vi "ToolBarButtonDraw.vi"(8 "error in (no error)":errorcluster, 9 "Coords":T1, 11 "Gviewer in":refnum<class "Gviewer.lvclass">) -> (0 "error out":errorcluster, 3 "Gviewer out":refnum<class "Gviewer.lvclass">)   [LabVIEW 2020, in "Sgraph_lib_V1.lvlib" / "Gviewer.lvclass"]
doc: "Draw toolbar buttons and objects on mouse move"
uses:
  Gviewer.lvclass
  <vilib>/Utility/miscctls.llb/LVPoint32TypeDef.ctl
  Gviewer.lvclass/Gviewer.ctl
  controls/AutoScale.ctl
  Common/controls/ToolTypeEnum.ctl
  Builds/Sgraph_lib_V1.lvlib
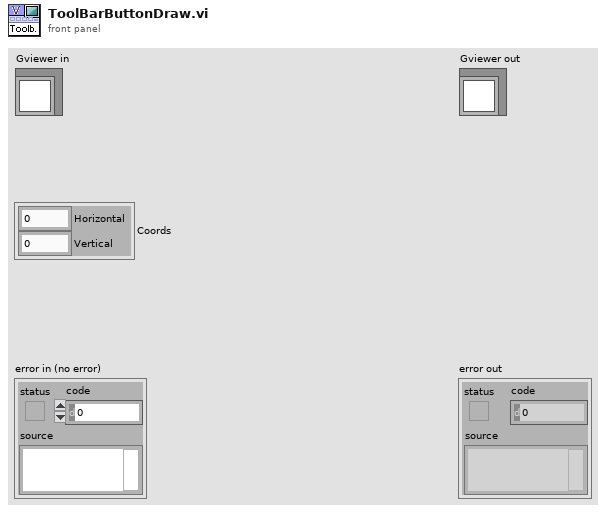
[diagram p1: front panel]
types:
  T1 = typedef "LVPoint32TypeDef.ctl" = cluster{"Horizontal":i32, "Vertical":i32}
  T2 = cluster{"left":i16, "top":i16, "right":i16, "bottom":i16}
  T3 = cluster{"horizontal":enum16{"left", "center", "right"}, "vertical":enum16{"top", "center", "bottom"}}
  T4 = typedef "Sgraph_lib_V1.lvlib/Gviewer.lvclass/AutoScale.ctl" = enum16{"FitEqual", "FitMax", "StackEqual", "StackMax", "StackPerType"}
  T5 = typedef "Sgraph_lib_V1.lvlib/Gviewer.lvclass/Typedef_ZoomEvent.ctl" = cluster{"Time-Start":timestamp, "Time-End":timestamp, "TimeSpan(sec)":dbl, "Live":T6, "SelProperties":T7[], "Time Stamp":timestamp}
  T6 = typedef "Sgraph_lib_V1.lvlib/Gviewer.lvclass/Typedef_Live.ctl" = enum16{"Live View", "Freeze"}
  T7 = typedef "Sgraph_lib_V1.lvlib/Gviewer.lvclass/Typedef_SelProperties.ctl" = cluster{"Color":u32, "LineType":T8, "max":dbl, "min":dbl}
  T8 = typedef "Sgraph_lib_V1.lvlib/Gviewer.lvclass/Typedef_LineType.ctl" = enum16{"num_bare", "num_MinMax_Area", "num_MinMax_Lines", "num_MinMax_Forfor", "num_Max_Area", "num_Max_Line", "num_Max_Forfor", "num_Min_Area", "num_Min_Line", "num_Min_Fosfor", "Boolean_Line_01", "Boolean_Area_01", "Boolean_Fosfor_01", "Boolean_Line_TF", "Boolean_Area_TF", "Boolean_Fosfor_TF", "Boolean_OnOff_Line", "Boolean_OnOff_Area", "Boolean_OnOff_Fosfor", "Boolean_spare", "StringEvent_Line", "StringEvent_TimeLine"}
  T9 = typedef "Sgraph_lib_V1.lvlib/ToolTypeEnum.ctl" = enum16{"00_Esc button", "01_Undo", "02_HelpButton", "03_CursorViewButton", "04_AutoScale_Fit", "05_AutoScale_Stacked", "06_ZoomWindowStart", "07_ZoomTimeStart", "08_ZoomAmplitudeStart", "09", "10", "11", "12", "13", "14", "15", "16", "17", "18", "19", "20_VerticalScroll", "21_VerticalMove", "22_TimeScroll", "23_TimeMove", "24", "25", "26_ZoomWindowSize", "27_ZoomTimeWindowSize", "28_ZoomAmplitudeWindowSize", "29", "30_LegendMovePoint", "31_LegendMoveDrag", "32", "33", "34", "35", "36", "37", "38", "39", "40_AddYscalePoint", "41_AddYscalePlace", "42_AddYscaleMovePoint", "43_AddYscaleMoveDrag", "44_AddYscaleDeletePoint"}
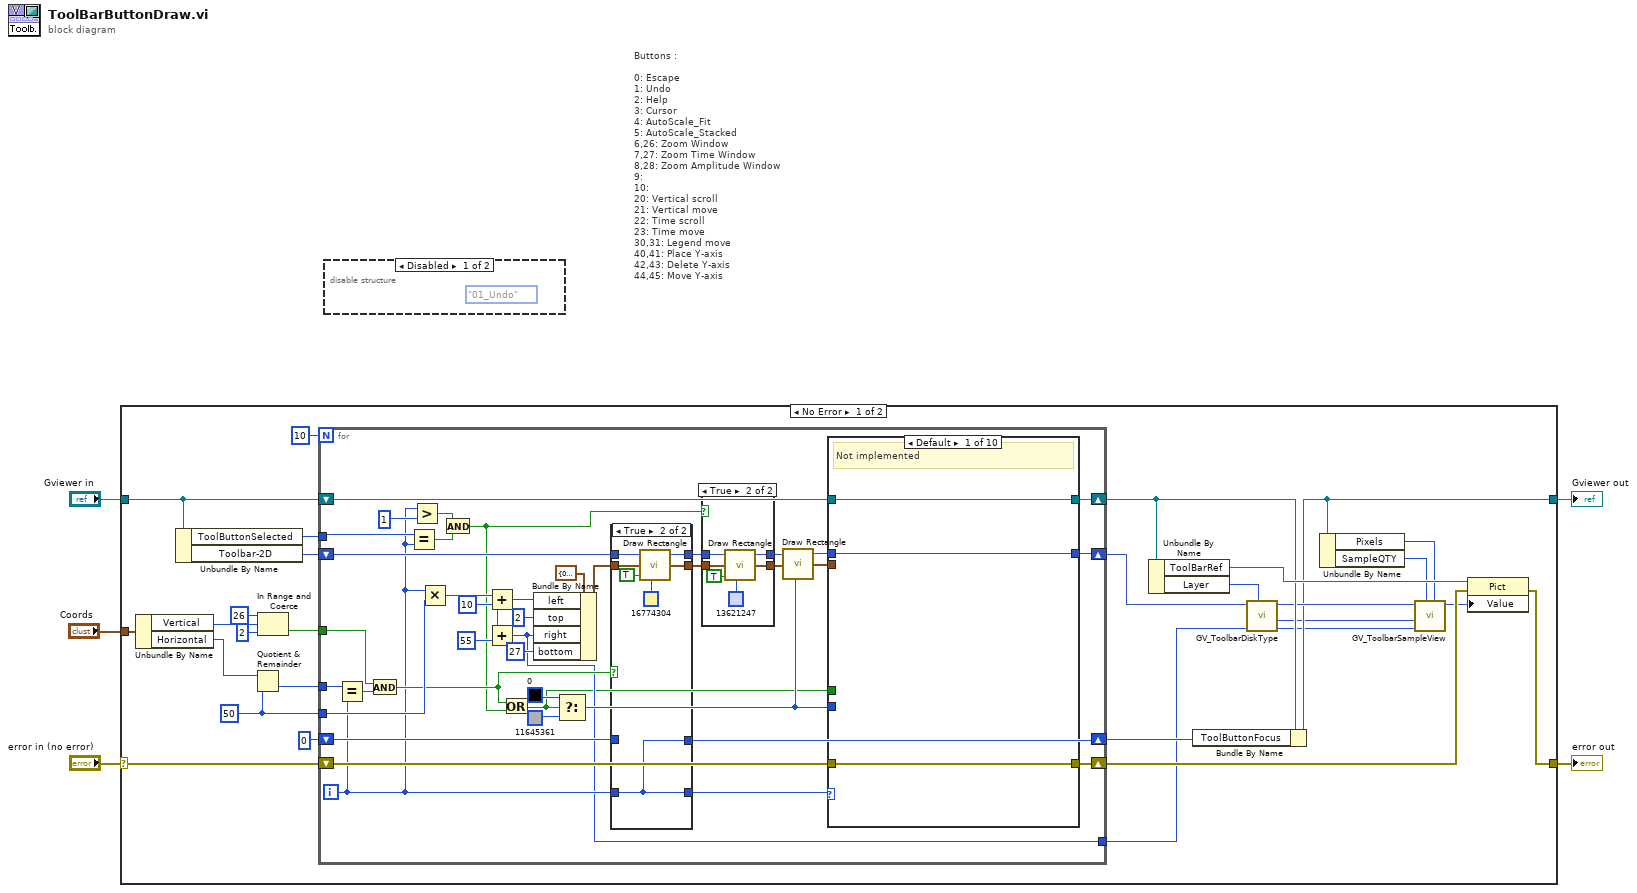
[diagram p0: block diagram]
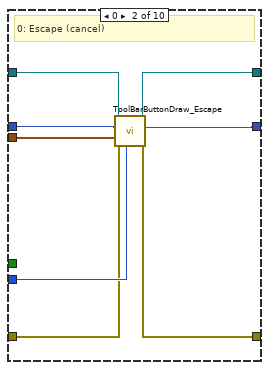
[diagram p3: hidden frame]
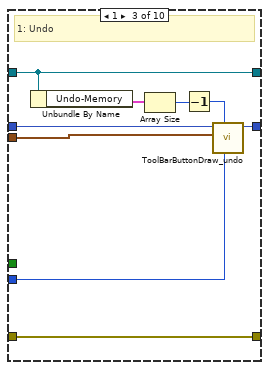
[diagram p4: hidden frame]
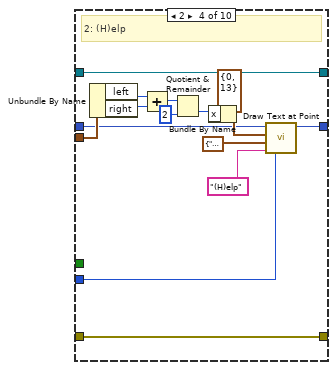
[diagram p5: hidden frame]
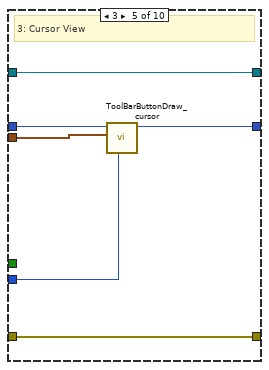
[diagram p6: hidden frame]
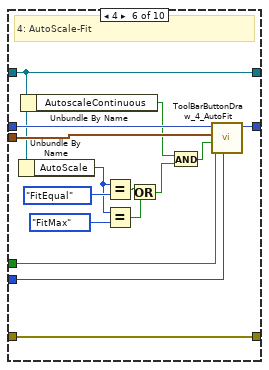
[diagram p7: hidden frame]
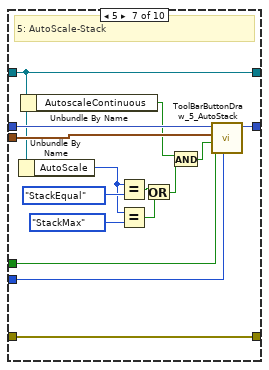
[diagram p8: hidden frame]
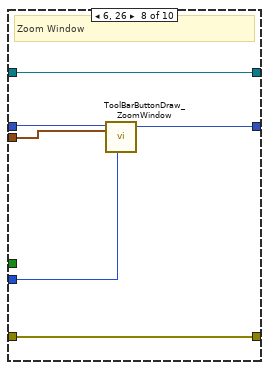
[diagram p9: hidden frame]
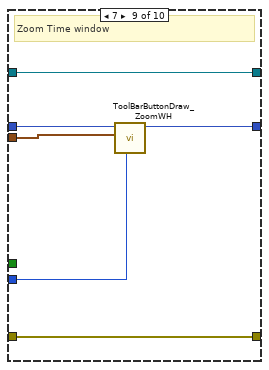
[diagram p10: hidden frame]
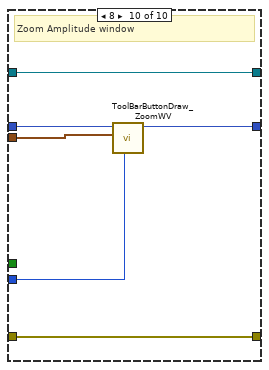
[diagram p11: hidden frame]
diagram:
  # "Buttons :\n\n0: Escape\n1: Undo\n2: Help\n3: Cursor\n4: AutoScale_Fit\n5: AutoScale_Stacked\n6,26: Zoom Window\n7,27: Zoom Time Window\n8,28: Zoom Amplitude Window\n9:\n10:\n20: Vertical scroll\n21: Vertical move\n22: Time scroll\n23: Time move\n30,31: Legend move\n40,41: Place Y-axis\n42,43: Delete Y-axis\n44,45: Move Y-axis"
  n1 = case shown="No Error" "error in (no error)" {
    selector: "error in (no error)" -> [w34 w180]
    tunnel: [w28 w180] -> w4
    tunnel: [w10 w179] -> w2
    tunnel: "Gviewer in" -> [w33 w179]
    tunnel: "Coords" -> [w27 _]
    frame No Error {
      w21 = 50 ("y")
      n2 = Unbundle By Name(w27) -> ("Vertical"=w26:i32, "Horizontal"=w22:i32)
      n3 = Unbundle By Name(w33) -> ("ToolButtonSelected"=w19:i32, "Toolbar-2D"=w32:picture)
      n4 = Quotient & Remainder(x=w22, y=w21) -> (floor(x/y)=w20:i32)  [unwired: 1 out]
      n5 = In Range and Coerce(upper limit=26, x=w26, lower limit=2) -> (In Range?=w23:bool)  [unwired: 1 out]
      n6 = for {
        N: 10 -> [_]
        shift-right: [w47] -> w16
        shift-left: w33 -> [w48]
        shift-right: [w43] -> w29
        shift-left: w34 -> [w44]
        shift-right: [w45] -> w15
        shift-left: w32 -> [w59]
        tunnel: w23 -> [w62]
        tunnel: w21 -> [w65]
        tunnel: w20 -> [w64]
        tunnel: w19 -> [w54]
        shift-right: [w40] -> w17
        shift-left: 0 -> [w41]
        tunnel: [w36] -> w11
        i -> [w39]
        n7 = Equal?(x=w64, y=w39) -> (x = y?=w63:bool)
        n8 = And(x=w62, y=w63) -> (x .and. y?=w50:bool)
        n9 = Equal?(x=w54, y=w39) -> (x = y?=w52:bool)
        n10 = Greater?(x=w39, y=1 ("x")) -> (0:w53:bool)
        n11 = Multiply(x=w39, y=w65) -> (x*y=w69:i32)
        n12 = And(x=w53, y=w52) -> (x .and. y?=w49:bool)
        n13 = Add(x=w69, y=10) -> (x+y=w66:i32)
        n14 = Add(x=w69, y=55) -> (x+y=w36:i32)
        n15 = Or(x=w50, y=w49) -> (x .or. y?=w35:bool)
        n16 = Bundle By Name(cluster=T2 {"left"=0, "top"=0, "right"=0, "bottom"=0} ("rect"), "left"=w66, "top"=i16 2, "right"=w36, "bottom"=i16 27) -> (w58:T2)
        n17 = Select(t=u32 0, s=w35, f=u32 11645361) -> (s? t:f=w42:u32)
        n18 = case shown="True" w50 {
          tunnel: w59 -> [w172 w178]
          tunnel: [w172 w177] -> w57
          tunnel: w58 -> [w171 w176]
          tunnel: [w171 w176] -> w55
          tunnel: w41 -> [w170 _]
          tunnel: [w170 w173] -> w40
          tunnel: w39 -> [w169 w173]
          tunnel: [w169 w173] -> w38
          frame False {
          }
          frame True {
            n19 = call <vilib>:"Draw Rectangle.vi"("picture"=w178, "rect"=w176, "fill?(F)"=TRUE, "color(black)"=u32 16774304) -> ("new picture"=w177:picture)  [unwired: 5 in]
          }
        }
        n20 = case shown="True" w49 {
          tunnel: w57 -> [w163 w167]
          tunnel: [w163 w166] -> w56
          tunnel: w55 -> [w162 w168]
          tunnel: [w162 w168] -> w37
          frame False {
          }
          frame True {
            n21 = call <vilib>:"Draw Rectangle.vi"("picture"=w167, "rect"=w168, "fill?(F)"=TRUE, "color(black)"=u32 13621247) -> ("new picture"=w166:picture)  [unwired: 5 in]
          }
        }
        n22 = call <vilib>:"Draw Rectangle.vi"("picture"=w56, "rect"=w37, "color(black)"=w42) -> ("new picture"=w46:picture)  [unwired: 6 in]
        n23 = case shown="Default" w38 {
          tunnel: w48 -> [w75 w80 w87 w107 w113 w117 w132 w149 w155 w161]
          tunnel: [w75 w81 w87 w107 w113 w117 w132 w149 w155 w161] -> w47
          tunnel: w46 -> [w74 w77 w91 w93 w112 w128 w143 w147 w153 w159]
          tunnel: [w74 w76 w90 w105 w108 w124 w139 w146 w152 w158] -> w45
          tunnel: w44 -> [w73 w78 w92 w106 w109 w125 w140 w148 w154 w160]
          tunnel: [w73 w79 w92 w106 w109 w125 w140 w148 w154 w160] -> w43
          tunnel: w42 -> [_ w82 w88 w104 w110 w126 w141 w144 w150 w156]
          tunnel: w37 -> [_ w83 w89 w99 w111 w127 w142 w145 w151 w157]
          tunnel: w35 -> [_ _ _ _ _ w123 w138 _ _ _]
          frame Default {
            # "Not implemented"
          }
          frame 0 {
            # "0: Escape (cancel)"
            n24 = call "ToolBarButtonDraw_Escape.vi"("Color"=w82, "error in"=w78, "rect"=w83, "Pict IN"=w77, "Gviewer in"=w80) -> ("error out"=w79:errorcluster, "Pict OUT"=w76:picture, "Gviewer out"=w81:refnum<class "Gviewer.lvclass">)  [unwired: 4 in]
          }
          frame 1 {
            # "1: Undo"
            n25 = Unbundle By Name(w87) -> ("Undo-Memory"=w86:T5[])
            n26 = Array Size(array=w86) -> (size(s)=w85:i32)
            n27 = Decrement(x=w85) -> (x-1=w84:i32)
            n28 = call "ToolBarButtonDraw_undo.vi"("Color"=w88, "undo size"=w84, "rect"=w89, "Pict IN"=w91) -> ("Pict OUT"=w90:picture)  [unwired: 7 in]
          }
          frame 2 {
            # "2: (H)elp"
            n29 = Unbundle By Name(w99) -> ("left"=w98:i16, "right"=w97:i16)
            n30 = Add(x=w98, y=w97) -> (x+y=w96:i16)
            n31 = Quotient & Remainder(x=w96, y=i16 2) -> (floor(x/y)=w94:i16)  [unwired: 1 out]
            n32 = Bundle By Name(cluster=cluster{"x":i16, "y":i16} {"x"=0, "y"=13} ("origin"), "x"=w94) -> (w101:cluster{"x":i16, "y":i16})
            n33 = call <vilib>:"Draw Text at Point.vi"("text color(black)"=w104, "text"="(H)elp", "alignment(left, top)"=T3 {"horizontal"=enum."center", "vertical"=enum."center"}, "origin"=w101, "picture"=w93) -> ("new picture"=w105:picture)  [unwired: 5 in, 1 out]
          }
          frame 3 {
            # "3: Cursor View"
            n34 = call "ToolBarButtonDraw_cursor.vi"("Color"=w110, "rect"=w111, "Pict IN"=w112) -> ("Pict OUT"=w108:picture)  [unwired: 8 in]
          }
          frame 4 {
            # "4: AutoScale-Fit"
            n35 = Unbundle By Name(w117) -> ("AutoScale"=w121:T4)
            n36 = Unbundle By Name(w117) -> ("AutoscaleContinuous"=w116:bool)
            n37 = Equal?(x=w121, y=AutoScale."FitEqual" ("AutoScale")) -> (x = y?=w119:bool)
            n38 = Equal?(x=w121, y=AutoScale."FitMax" ("AutoScale")) -> (x = y?=w118:bool)
            n39 = Or(x=w119, y=w118) -> (x .or. y?=w115:bool)
            n40 = And(x=w116, y=w115) -> (x .and. y?=w114:bool)
            n41 = call "ToolBarButtonDraw_4_AutoFit.vi"("Color"=w126, "Focus"=w123, "Continuous"=w114, "rect"=w127, "Pict IN"=w128) -> ("Pict OUT"=w124:picture)  [unwired: 6 in]
          }
          frame 5 {
            # "5: AutoScale-Stack"
            n42 = Unbundle By Name(w132) -> ("AutoScale"=w136:T4)
            n43 = Unbundle By Name(w132) -> ("AutoscaleContinuous"=w131:bool)
            n44 = Equal?(x=w136, y=AutoScale."StackEqual" ("AutoScale")) -> (x = y?=w134:bool)
            n45 = Equal?(x=w136, y=AutoScale."StackMax" ("AutoScale")) -> (x = y?=w133:bool)
            n46 = Or(x=w134, y=w133) -> (x .or. y?=w130:bool)
            n47 = And(x=w131, y=w130) -> (x .and. y?=w129:bool)
            n48 = call "ToolBarButtonDraw_5_AutoStack.vi"("Color"=w141, "Focus"=w138, "Continuous"=w129, "rect"=w142, "Pict IN"=w143) -> ("Pict OUT"=w139:picture)  [unwired: 6 in]
          }
          frame 6, 26 {
            # "Zoom Window"
            n49 = call "ToolBarButtonDraw_ZoomWindow.vi"("Color"=w144, "rect"=w145, "Pict IN"=w147) -> ("Pict OUT"=w146:picture)  [unwired: 8 in]
          }
          frame 7 {
            # "Zoom Time window"
            n50 = call "ToolBarButtonDraw_ZoomWH.vi"("Color"=w150, "rect"=w151, "Pict IN"=w153) -> ("Pict OUT"=w152:picture)  [unwired: 8 in]
          }
          frame 8 {
            # "Zoom Amplitude window"
            n51 = call "ToolBarButtonDraw_ZoomWV.vi"("Color"=w156, "rect"=w157, "Pict IN"=w159) -> ("Pict OUT"=w158:picture)  [unwired: 8 in]
          }
        }
      }
      n52 = Unbundle By Name(w16) -> ("ToolBarRef"=w30:refnum<vi>, "Layer"=w14:i32)
      n53 = Bundle By Name(cluster=w16, "ToolButtonFocus"=w17) -> (w10:refnum<class "Gviewer.lvclass">)
      n54 = call "GV_ToolbarDiskType.vi"("Layer"=w14, "Hor-pos"=w11, "Pict in"=w15) -> ("x"=w7:i16, "y"=w8:i16, "Pict out"=w13:picture)  [unwired: 6 in]
      n55 = Unbundle By Name(w10) -> ("Pixels"=w6:i32, "SampleQTY"=w9:i32)
      n56 = call "GV_ToolbarSampleView.vi"("Pixels"=w6, "Samples"=w9, "Hor-pos"=w7, "y"=w8, "Pict in"=w13) -> ("Pict out"=w12:picture)  [unwired: 6 in]
      n57 = property class="Pict"(reference=w30, error in=w29, "Value"=w12) -> (error out=w28:errorcluster)  [unwired: 1 out]
    }
    frame Error {
    }
  }
  "error out" <- w4
  "Gviewer out" <- w2
  n58 = disable-structure shown="Disabled" {
    frame Disabled {
      (unwired) ToolTypeEnum."01_Undo" ("Enum")
    }
    frame Enabled {
    }
  }
